vi "Create.vi"(10 "JSON Charting Config":T1) -> (3 "Charting Config Value out":refnum<class "Charting Config Value.lvclass">)   [LabVIEW 2020, in "VolatusGUI.lvlib" / "Charting Config Value.lvclass"]
uses:
  Charting Config Value.lvclass
  Charting Config Value.lvclass/Charting Config Value.ctl
  Historian Charting Manager/JSON Chart Group.ctl
  VolatusGUI.lvlib
  Historian Charting Manager/JSON Plot Config.ctl
  Historian Charting Manager/JSON Plot Group.ctl
  Historian Charting Manager/JSON Charting Config.ctl
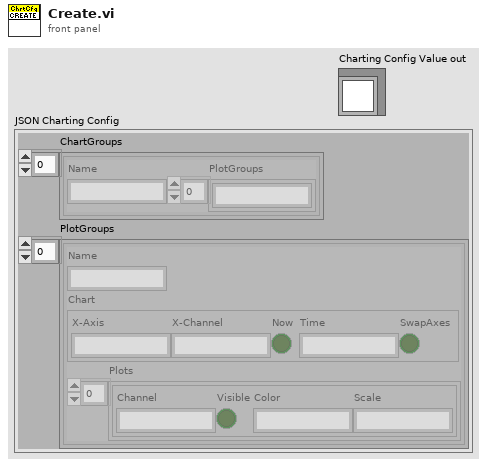
[diagram p1: front panel]
types:
  T1 = typedef "VolatusGUI.lvlib/JSON Charting Config.ctl" = cluster{"ChartGroups":T2[], "PlotGroups":T3[]}
  T2 = typedef "VolatusGUI.lvlib/JSON Chart Group.ctl" = cluster{"Name":string, "PlotGroups":string[]}
  T3 = typedef "VolatusGUI.lvlib/JSON Plot Group.ctl" = cluster{"Name":string, "Chart":cluster{"X-Axis":string, "X-Channel":string, "Now":bool, "Time":string, "SwapAxes":bool}, "Plots":T4[]}
  T4 = typedef "VolatusGUI.lvlib/JSON Plot Config.ctl" = cluster{"Channel":string, "Visible":bool, "Color":string, "Scale":string}
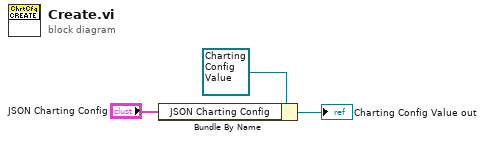
[diagram p0: block diagram]
diagram:
  n1 = Bundle By Name(cluster=refnum<class "Charting Config Value.lvclass"> refnum ("Charting Config Value in"), "JSON Charting Config"="JSON Charting Config") -> (→"Charting Config Value out":refnum<class "Charting Config Value.lvclass">)
